vi "Test Display.vi"(8 "error in (no error)":errorcluster, 10 "state":u16(ring) items=["off", "on"], 11 "VGC in":refnum<class "PL Inficon VGC.lvclass">) -> (0 "error out":errorcluster, 2 "state":u16(ring) items=["off", "on"], 3 "VGC out":refnum<class "PL Inficon VGC.lvclass">)   [LabVIEW 2015, in "PL Inficon VGC.lvclass"]
doc: "Tests display."
uses:
  PL Inficon VGC.lvclass
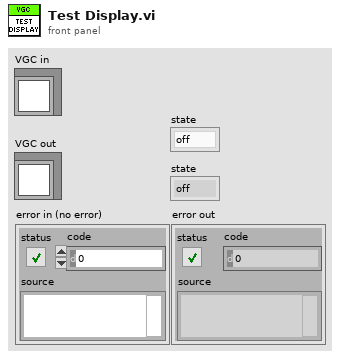
[diagram p1: front panel]
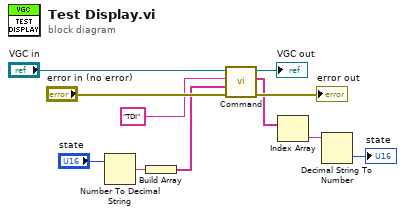
[diagram p0: block diagram]
diagram:
  n1 = Number To Decimal String(number="state") -> (decimal integer string=w2:string)  [unwired: 1 in]
  n2 = Build Array(w2) -> (w1:string[])
  n3 = call "Command.vi"("error in (no error)"="error in (no error)", "parameters"=w1, "command"="TDI", "VGC in"="VGC in") -> ("error out"=→"error out":errorcluster, "response data"=w6:string[], "VGC out"=→"VGC out":refnum<class "PL Inficon VGC.lvclass">)  [unwired: 5 in]
  n4 = Index Array(array=w6) -> (element=w5:string)  [unwired: 1 in]
  n5 = Decimal String To Number(string=w5) -> (number=→"state":i32)  [unwired: 2 in, 1 out]
